vi "Initialize.vi"(0 "PDF Table Class in":refnum<class "Pdfp Table Class.lvclass">, 11 "error in (no error)":errorcluster) -> (4 "PDF Table Class out":refnum<class "Pdfp Table Class.lvclass">, 15 "error out":errorcluster)   [LabVIEW 2020, in "Exaprom PDF.lvlib" / "Pdfp Table Class.lvclass"]
uses:
  <userlib>/labview-PDF-writer-master/LV Class/Pdfp Table Class/Pdfp Table Class.lvclass
  <userlib>/labview-PDF-writer-master/Controls/Table Controls/Table properties.ctl
  <userlib>/labview-PDF-writer-master/Controls/Table Controls/Table position.ctl
  <userlib>/labview-PDF-writer-master/Controls/Table Controls/Table type.ctl
  <userlib>/labview-PDF-writer-master/Controls/General Controls/Image to Add [ ].ctl
  <userlib>/labview-PDF-writer-master/Controls/Image Controls/Image Scale.ctl
  <userlib>/labview-PDF-writer-master/Controls/Table Controls/Table Appearance and Font Row [ ].ctl
  <userlib>/labview-PDF-writer-master/Controls/Table Controls/One Row Appearance.ctl
  <userlib>/labview-PDF-writer-master/Controls/Table Controls/Row from to.ctl
  <userlib>/labview-PDF-writer-master/Controls/Table Controls/Cell, Alignment, LS and Font - hide Vmerge.ctl
  <userlib>/labview-PDF-writer-master/Controls/Table Controls/Cell Type, Alignment and LS.ctl
  <userlib>/labview-PDF-writer-master/Controls/Table Controls/Cell Alignment 20px.ctl
  <userlib>/labview-PDF-writer-master/Controls/Table Controls/Text vertical arrangement.ctl
  <userlib>/labview-PDF-writer-master/Controls/Text Controls/Line spacing.ctl
  <userlib>/labview-PDF-writer-master/Controls/Table Controls/Cell Appearance.ctl
  <userlib>/labview-PDF-writer-master/Controls/Table Controls/Cell Border 20 px.ctl
  <userlib>/labview-PDF-writer-master/Controls/Table Controls/Merge Horizontal.ctl
  <userlib>/labview-PDF-writer-master/Controls/Table Controls/Merge Vertical.ctl
  <userlib>/labview-PDF-writer-master/Controls/Font Controls/Font complete cluster.ctl
  <userlib>/labview-PDF-writer-master/Controls/Font Controls/Font size.ctl
  <userlib>/labview-PDF-writer-master/Controls/Font Controls/Font color.ctl
  <userlib>/labview-PDF-writer-master/Controls/Font Controls/Type and encoding.ctl
  <userlib>/labview-PDF-writer-master/Controls/Text Controls/Unicode/Type and run direction.ctl
  <userlib>/labview-PDF-writer-master/Controls/Initialization Controls/Defaut Paragraphe and Line Spacing.ctl
  <userlib>/labview-PDF-writer-master/Controls/Text Controls/Texte alignement.ctl
  <userlib>/labview-PDF-writer-master/Controls/Font Controls/System Fonts.ctl
  <userlib>/labview-PDF-writer-master/LV Class/Pdfp Table Class/Pdfp Table Class.lvclass/Pdfp Table Class.ctl
  C:/Program Files (x86)/National Instruments/LabVIEW 2020/user.lib/labview-PDF-writer-master/DLL/itextsharp.dll
  DLL/itextsharp.dll
  <userlib>/labview-PDF-writer-master/Exaprom PDF.lvlib
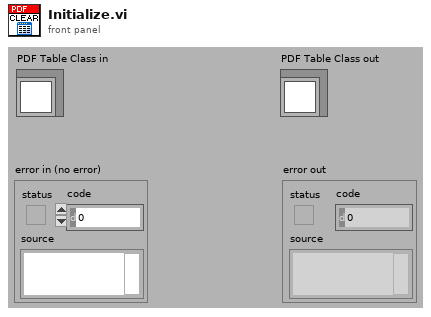
[diagram p1: front panel]
types:
  T1 = typedef "Exaprom PDF.lvlib/Defaut Paragraphe and Line Spacing.ctl" = cluster{" Aligment":T2, "Line spacing":T3}
  T2 = typedef "Exaprom PDF.lvlib/Texte alignement.ctl" = enum16{"Select", "CENTER", "JUSTIFY", "LEFT", "RIGHT"}
  T3 = typedef "Exaprom PDF.lvlib/Line spacing.ctl" = enum16{"Select", "1.0", "1.5", "2.0"}
  T4 = typedef "Exaprom PDF.lvlib/Font complete cluster.ctl" = cluster{"Name":string, "Size":T5, "Color":T6, "Style":cluster{"Bold":bool, "Italic":bool, "Underline":bool, "Strikeout":bool}, "Type":T7}
  T5 = typedef "Exaprom PDF.lvlib/Font size.ctl" = sgl
  T6 = typedef "Exaprom PDF.lvlib/Font color.ctl" = u32
  T7 = typedef "Exaprom PDF.lvlib/Type and encoding.ctl" = cluster{"Type&direction":T8, "Embedded":bool, "Encoding":string}
  T8 = typedef "Exaprom PDF.lvlib/Type and run direction.ctl" = enum16{"Select", "ASCII", "UTF-16", "UTF-16 (default)", "UTF-16 (LTR)", "UTF-16 (RTL)"}
  T9 = typedef "Exaprom PDF.lvlib/System Fonts.ctl" = cluster{"Font name [ ]":string[], "Font and file names [ ]":cluster{"Font name":string, "File name":string}[]}
  T10 = cluster{"Paragraphe cluster":T1, "Font":T4, "Font Ref":refnum<k24>, "System Fonts":T9}
  T11 = typedef "Exaprom PDF.lvlib/Table Appearance and Font Row [ ].ctl" = T12[]
  T12 = typedef "Exaprom PDF.lvlib/One Row Appearance.ctl" = cluster{"Row":T13, "Cell [ ]":T14[]}
  T13 = typedef "Exaprom PDF.lvlib/Row from to.ctl" = cluster{"From #":i16, "to #":i16}
  T14 = typedef "Exaprom PDF.lvlib/Cell, Alignment, LS and Font - hide Vmerge.ctl" = cluster{"Text":T15, "Cell Appearance":T18, "HMerge":T20, "VMerge":T21, "Font":T4}
  T15 = typedef "Exaprom PDF.lvlib/Cell Type, Alignment and LS.ctl" = cluster{"Cell Alignment":T16, "Text rotation":T17, "Line spacing":T3}
  T16 = typedef "Exaprom PDF.lvlib/Cell Alignment 20px.ctl" = u16
  T17 = typedef "Exaprom PDF.lvlib/Text vertical arrangement.ctl" = enum16{"None", "Clockwise", "Counterclockwise"}
  T18 = typedef "Exaprom PDF.lvlib/Cell Appearance.ctl" = cluster{"Border":T19, "Thickness":sgl, "Color":u32, "BG":u32}
  T19 = typedef "Exaprom PDF.lvlib/Cell Border 20 px.ctl" = u16
  T20 = typedef "Exaprom PDF.lvlib/Merge Horizontal.ctl" = cluster{"From":i8, "to":i8}
  T21 = typedef "Exaprom PDF.lvlib/Merge Vertical.ctl" = cluster{"From":i8, "to":i8}
  T22 = typedef "Exaprom PDF.lvlib/Image to Add [ ].ctl" = cluster{"Image name":string, "Path":path, "Scale":T23}[]
  T23 = typedef "Exaprom PDF.lvlib/Image Scale.ctl" = sgl
  T24 = typedef "Exaprom PDF.lvlib/Table type.ctl" = enum16{"Standard", "Customized"}
  T25 = typedef "Exaprom PDF.lvlib/Table properties.ctl" = cluster{"Table position":T26, "SpacingBefore (points)":sgl, "SpacingAfter (points)":sgl}
  T26 = typedef "Exaprom PDF.lvlib/Table position.ctl" = i32
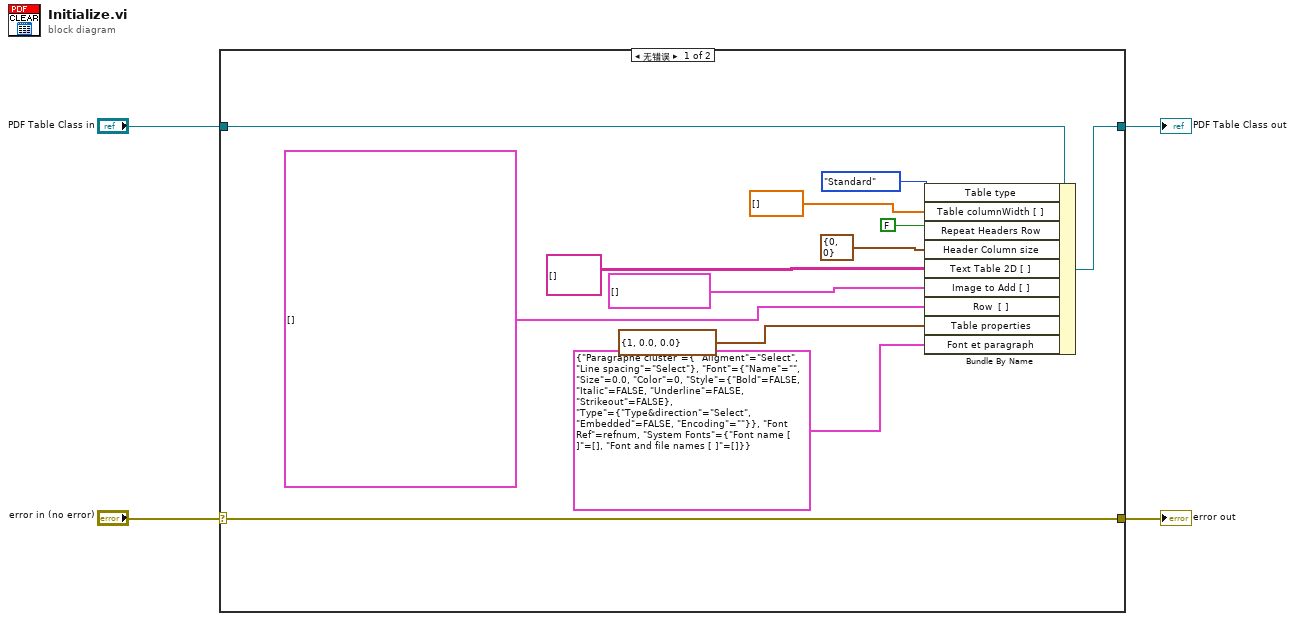
[diagram p0: block diagram]
diagram:
  n1 = case shown="无错误" "error in (no error)" {
    selector: "error in (no error)" -> [w16 w18]
    tunnel: [w16 w18] -> w3
    tunnel: [w14 w17] -> w1
    tunnel: "PDF Table Class in" -> [w15 w17]
    frame No Error {
      n2 = Bundle By Name(cluster=w15, "Table type"=Table_type."Standard", "Table columnWidth [ ]"=sgl[] [], "Repeat Headers Row"=FALSE, "Header Column size"=cluster{"# Column":u16, "# Row":u16} {"# Column"=0, "# Row"=0}, "Text Table 2D [ ]"=string[][] [], "Image to Add [ ]"=T22 [], "Row  [ ]"=T11 [], "Table properties"=T25 {"Table position"=1, "SpacingBefore (points)"=0.0, "SpacingAfter (points)"=0.0}, "Font et paragraph"=T10 {"Paragraphe cluster"={" Aligment"=enum."Select", "Line spacing"=enum."Select"}, "Font"={"Name"="", "Size"=0.0, "Color"=0, "Style"={"Bold"=FALSE, "Italic"=FALSE, "Underline"=FALSE, "Strikeout"=FALSE}, "Type"={"Type&direction"=enum."Select", "Embedded"=FALSE, "Encoding"=""}}, "Font Ref"=refnum, "System Fonts"={"Font name [ ]"=[], "Font and file names [ ]"=[]}}) -> (w14:refnum<class "Pdfp Table Class.lvclass">)
    }
    frame Error {
    }
  }
  "error out" <- w3
  "PDF Table Class out" <- w1
